vi "PositionOpenClose.vi"   [LabVIEW 2016, in "Gear Manipulator.lvclass"]
uses:
  Gear Manipulator.lvclass
  Gear Manipulator.lvclass/Gear Manipulator.ctl
  <vilib>/Rock Robotics/WPI/Solenoid/WPI_SolenoidValue.ctl
  <vilib>/Rock Robotics/WPI/Solenoid/WPI_SolenoidSetEnum.vi
types:
  T1 = typedef "WPI_SolenoidValue.ctl" = enum16{"Off", "On", "Forward", "Reverse"}
  T2 = typedef "WPI_SolenoidDevRef.ctl" = cluster{"DevStatus":errorcluster, "Pneumatics Control Module":u8, "Forward Solenoid Channel":T3, "Reverse Solenoid Channel":T3}
  T3 = typedef "WPI_SolenoidChannel.ctl" = enum8{"Solenoid 0", "Solenoid 1", "Solenoid 2", "Solenoid 3", "Solenoid 4", "Solenoid 5", "Solenoid 6", "Solenoid 7", "Invalid"}
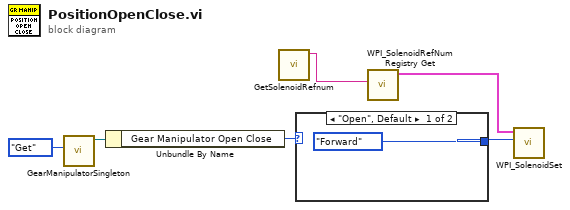
[diagram p0: block diagram]
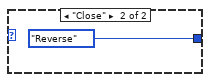
[diagram p2: hidden frame]
diagram:
  n1 = call "GearManipulatorSingleton.vi"("Get/Set"=enum16{"Get", "Set"}."Get") -> ("Gear Manipulator.lvclass"=w3:refnum<class "Gear Manipulator.lvclass">)  [unwired: 9 in, 1 out]
  n2 = Unbundle By Name(w3) -> ("Gear Manipulator Open Close"=w5:enum16{"Open", "Close"})
  n3 = call "GetSolenoidRefnum.vi"() -> ("OpenCloseSolenoidRefnum"=w1:string)  [unwired: 10 in, 1 out]
  n4 = case shown="\"Open\", Default" w5 {
    tunnel: [WPI_SolenoidValue."Forward" ("Value") WPI_SolenoidValue."Reverse" ("Value")] -> w6
    frame "Open", Default {
    }
    frame "Close" {
    }
  }
  n5 = call <vilib>:"WPI_SolenoidRefNum Registry Get.vi"("refnum name"=w1) -> ("SolenoidDevRef"=w2:T2)  [unwired: 9 in, 1 out]
  n6 = call-poly <vilib>:"WPI_SolenoidSet.vi"("Value"=w6, "SolenoidDevRef"=w2) -> ()  [unwired: 8 in, 2 out]
